vi "Get SLSC Module Resource.vi"(8 "error in (no error)":errorcluster, 11 "SLSC Module":T1 format="%.0x") -> (0 "error out":errorcluster, 2 "SLSC Module Resource":refnum<k21>, 3 "SLSC Module out":T1 format="%.0x")   [LabVIEW 2017, in "VeriStand SLSC Scripting.lvlib"]
uses:
  VeriStand SLSC Scripting.lvlib
  <vilib>/NI Veristand/Custom Device API/Custom Device Item Ref.ctl
  <vilib>/NI Veristand/Custom Device API/Get Item Property (I32).vi
  <vilib>/nisyscfg/Close (System).vi
  <vilib>/SLSC/Initialize Session with Devices.vi
  <vilib>/SLSC/Close Session.vi
  <vilib>/nisyscfg/nisyscfg.lvlib
  <resource>/objmgr/nisysapi.rc
  <vilib>/SLSC/SLSC.lvlib
  <resource>/objmgr/slsc.rc
  <vilib>/NI Veristand/Custom Device API/Custom Device API.lvlib
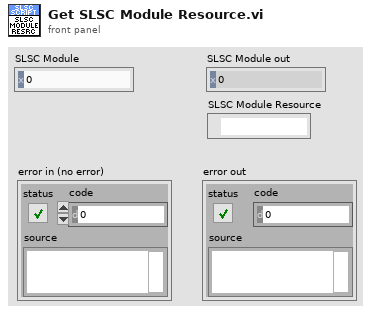
[diagram p1: front panel]
types:
  T1 = typedef "Custom Device API.lvlib/Custom Device Item Ref.ctl" = u64
  T2 = typedef "VeriStand SLSC Scripting.lvlib/SLSC Chassis ID.ctl" = cluster{"Name or IP":string, "ChassisIDType":i32, "chassisType":i32}
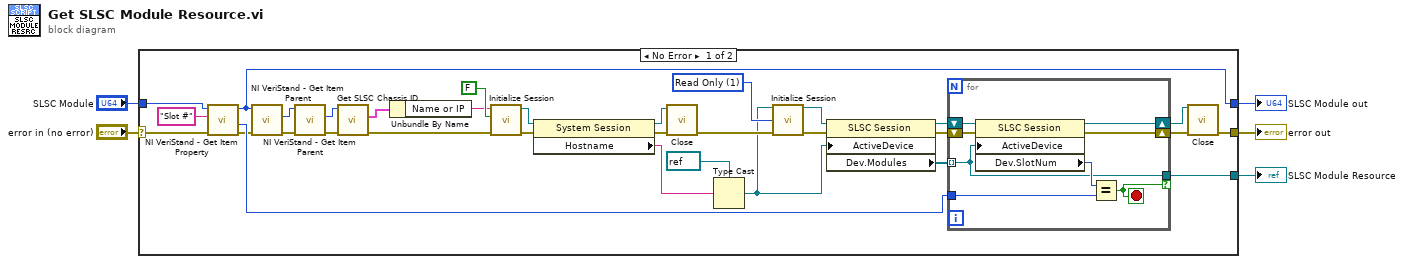
[diagram p0: block diagram]
diagram:
  n1 = case shown="No Error" "error in (no error)" {
    selector: "error in (no error)" -> [w23 w47]
    tunnel: [w21 _] -> w4
    tunnel: "SLSC Module" -> [w20 w46]
    tunnel: [w17 w47] -> w2
    tunnel: [w10 w46] -> w1
    frame No Error {
      w32 = 1 items=["None"=0, "Read Only"=1, "Read/Write"=3] ("reservation access (Read/Write)")
      n2 = call-poly <vilib>:"NI VeriStand - Get Item Property.vi"("error in (no error)"=w23, "Property Name"="Slot #", "Item Ref in"=w20) -> ("error out"=w11:errorcluster, "Value"=w22:i32, "Item Ref out"=w10:T1)  [unwired: 5 in, 1 out]
      n3 = call <vilib>:"NI VeriStand - Get Item Parent.vi"("error in (no error)"=w11, "Item Ref in"=w10) -> ("error out"=w12:errorcluster, "Parent Ref"=w9:T1)  [unwired: 6 in, 2 out]
      n4 = call <vilib>:"NI VeriStand - Get Item Parent.vi"("error in (no error)"=w12, "Item Ref in"=w9) -> ("error out"=w13:errorcluster, "Parent Ref"=w8:T1)  [unwired: 6 in, 2 out]
      n5 = call "Get SLSC Chassis ID.vi"("error in (no error)"=w13, "SLSC Chassis Ref in"=w8) -> ("error out"=w16:errorcluster, "SLSC Chassis ID"=w7:T2)  [unwired: 7 in, 1 out]
      n6 = Unbundle By Name(w7) -> ("Name or IP"=w6:string)
      n7 = call <vilib>:"Initialize Session.vi"("error in (no error)"=w16, "Force Property Refresh (T)"=FALSE, "Target (localhost)"=w6) -> ("error out"=w36:errorcluster, "Session out"=w37:refnum<k21>)  [unwired: 7 in]
      n8 = property class="System Session"(reference=w37, error in=w36) -> (reference out=w33:refnum<k21>, error out=w35:errorcluster, "Hostname"=w15:string)
      n9 = call-poly <vilib>:"Close.vi"("error in (no error)"=w35, "Session in"=w33) -> ("error out"=w31:errorcluster)  [unwired: 9 in]
      n10 = Type Cast(type=refnum<k21> refnum ("devices"), x=w15) -> (*(type *) &x=w27:refnum<k21>)
      n11 = call-poly <vilib>:"Initialize Session.vi"("devices"=w27, "reservation access (Read/Write)"=w32, "error in (no error)"=w31) -> ("session out"=w30:refnum<k21>, "error out"=w29:errorcluster)  [unwired: 11 in]
      n12 = property class="SLSC Session"(reference=w30, error in=w29, "ActiveDevice"=w27) -> (reference out=w26:refnum<k21>, error out=w25:errorcluster, "Dev.Modules"=w14:refnum<k21>[])
      n13 = for {
        tunnel: w14 -> [w39] mode=indexing
        shift-right: [w43] -> w18
        shift-left: w25 -> [w44]
        shift-right: [w42] -> w19
        shift-left: w26 -> [w45]
        tunnel: w22 -> [w40]
        tunnel: [w39] -> w21 if=w38
        stop <- w38 stop-if-true
        n14 = property class="SLSC Session"(reference=w45, error in=w44, "ActiveDevice"=w39) -> (reference out=w42:refnum<k21>, error out=w43:errorcluster, "Dev.SlotNum"=w41:u32)
        n15 = Equal?(x=w41, y=w40) -> (x = y?=w38:bool)
      }
      n16 = call-poly <vilib>:"Close.vi"("session in"=w19, "error in (no error)"=w18) -> ("error out"=w17:errorcluster)  [unwired: 13 in]
    }
    frame Error {
    }
  }
  "SLSC Module Resource" <- w4
  "SLSC Module out" <- w1
  "error out" <- w2
